vi "InitPID.vi"(4 "Side":enum16{"Load", "Drive"}(ring), 6 "Controller":T1(ring), 7 "PIDAdj":refnum<vi>, 8 "error in (no error)":errorcluster, 9 "refPIDProcessValue":refnum<vi>, 10 "refPIDSettingValue":refnum<vi>, 11 "PID in":refnum<class "PID.lvclass">) -> (0 "error out":errorcluster, 3 "PID out":refnum<class "PID.lvclass">)   [LabVIEW 2024, in "PID Actor.lvlib" / "PID.lvclass"]
uses:
  PID.lvclass
  PID.lvclass/PID.ctl
panel:
  in  "PIDAdj":T2={"PID Mode"=enum."Torque", "NP"=100.0, "NI"=100.0, "ND"=100.0, "NPS"="", "NIS"="", "NDS"=""} caption="PID Adj" {"ND" max=99.0; "NI" max=99.0 step=1.0; "NP" max=99.0}
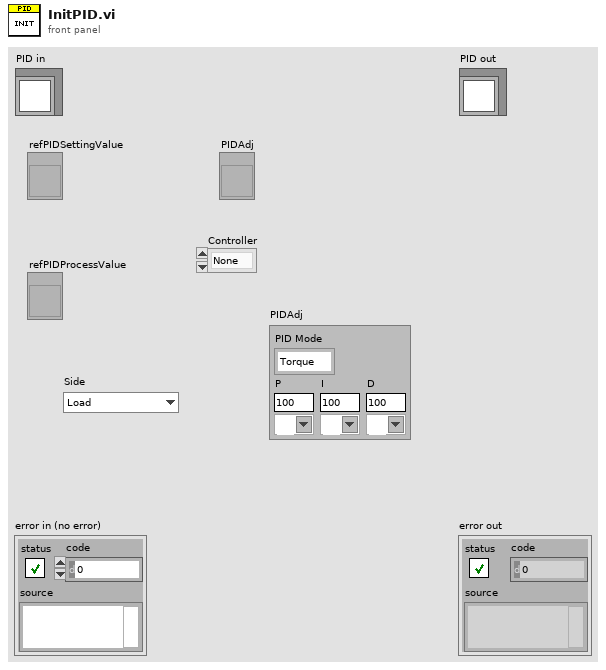
[diagram p1: front panel]
types:
  T1 = enum16{"None", "DSP 6001", "DSP 7000", "DC 2000", "DC 1000-A1", "DC 1000-S1", "DC 1000-S2", "DC 1000-S3", "DC 1000-S4", "DC 1500"}
  T2 = cluster{"PID Mode":enum16{"Torque", "Speed", "Ramp", "Amp", "Watts In", "Watts Out"}, "NP":dbl, "NI":dbl, "ND":dbl, "NPS":string, "NIS":string, "NDS":string}
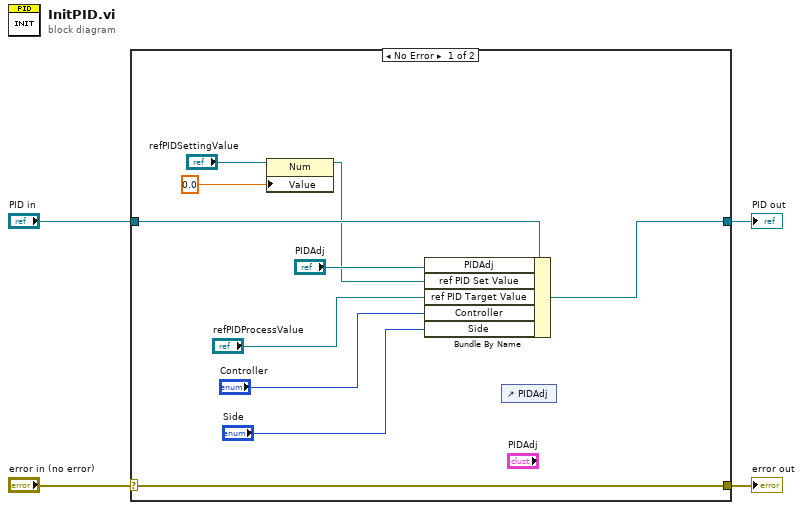
[diagram p0: block diagram]
diagram:
  n1 = case shown="No Error" "error in (no error)" {
    selector: "error in (no error)" -> [w14 w16]
    tunnel: [w14 w16] -> w3
    tunnel: [w8 w15] -> w1
    tunnel: "PID in" -> [w9 w15]
    frame No Error {
      n2 = property class="Num"(reference="refPIDSettingValue", "Value"=0.0) -> (reference out=w5:refnum<vi>)  [unwired: 1 in, 1 out]
      n3 = Bundle By Name(cluster=w9, "PIDAdj"="PIDAdj", "ref PID Set Value"=w5, "ref PID Target Value"="refPIDProcessValue", "Controller"="Controller", "Side"="Side") -> (w8:refnum<class "PID.lvclass">)
      n4 = control-ref of="PIDAdj"() -> ()  [unwired: 1 out]
    }
    frame Error {
    }
  }
  "error out" <- w3
  "PID out" <- w1
